vi "Encoder Math 2 no timing.vi"(0 "Encoder B":bool, 5 "Encoder A":bool, 7 "Encoder Reading":i32, 9 "Encoder A Old":bool, 11 "Encoder B Old":bool, 12 "Use Index to reset":bool, 13 "Encoder Index":bool) -> (4 "The Encoder Changed":bool, 6 "Count Zeroed at Index":i32, 8 "Encoder A Old (sReg)":bool, 10 "Encoder B Old (sReg)":bool, 14 "Current count Before Zeroing":i32, 15 "Resetting to zero":bool)   [LabVIEW 2009]
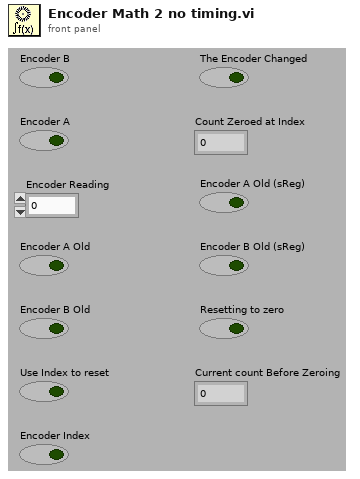
[diagram p1: front panel]
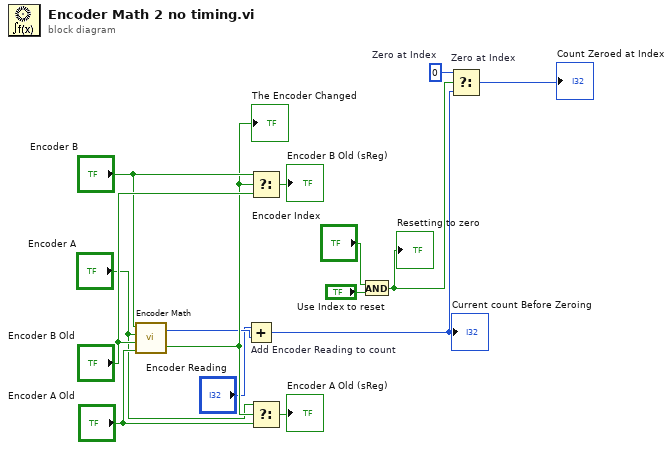
[diagram p0: block diagram]
diagram:
  w5 = 0  # Zero at Index
  n1 = call "Encoder Math.vi"("Encoder A_old"="Encoder A Old", "Encoder B_old"="Encoder B Old", "Encoder A_new"="Encoder A", "Encoder B_new"="Encoder B") -> ("The Encoder Changed"=w12:bool, "Change in Encoder Value"=w2:i32)
  "The Encoder Changed" <- w12
  n2 = Add "Add Encoder Reading to count"(x="Encoder Reading", y=w2) -> (x+y=w3:i32)
  "Current count Before Zeroing" <- w3
  n3 = Select(t="Encoder B", s=w12, f="Encoder B Old") -> (s? t:f=→"Encoder B Old (sReg)":bool)
  n4 = Select(t="Encoder A", s=w12, f="Encoder A Old") -> (s? t:f=→"Encoder A Old (sReg)":bool)
  n5 = And(x="Encoder Index", y="Use Index to reset") -> (x .and. y?=w8:bool)
  "Resetting to zero" <- w8
  n6 = Select "Zero at Index"(t=w5, s=w8, f=w3) -> (s? t:f=→"Count Zeroed at Index":i32)
